vi "TEST_ProcessData.vi"() -> ()   [LabVIEW 2024]
doc: "This VI is used to test the Spec LUT (Look Up Table) Select ChA!ChB and Drain!Fill\nShould produce the spec index for the level entered.\nNote: Meausre shows the value whre Measure R is enabled."
uses:
  Control Definitions/Def FullCfg.ctl
  Control Definitions/Def BenchCfg.ctl
  Control Definitions/Def PumpCtlRefs.ctl
  Control Definitions/Def_PumpSpeed.ctl
  Control Definitions/Def Bench Status.ctl
  Control Definitions/Def_LevelSwitched.ctl
  Control Definitions/Def Spec RNG.ctl
  Control Definitions/Ded LUT_Status.ctl
  Control Definitions/Def Results2.ctl
  Control Definitions/Def_ATPStatus.ctl
panel:
  out "L Err Num":i32
  out "R Err Num":i32
  in  "ATP Check":bool
  out "Results out":T1 {"Resistor" format="%.1f"; "Drain" format="%.3f"; "Fill" format="%.3f"}
  out "element":T3={"Specs"=[8.5, 8.5, 0.0, 102.0, 98.0, 0.0, 0.0], "LUT Status"={"ChA/!ChB"=TRUE, "Drain/!Fill"=FALSE, "In Range?"=FALSE, "Switch Range?"=FALSE, "Measure R?"=FALSE, "Vaild R?"=FALSE, "Index(n)"=0, "Index(n)-1"=-1, "Index Max"=13, "Index(n-1)"=0}}
  out "Level Out":T5={"Switched"=FALSE, "Level OUt"=8.030499999999925, "Double Err"=FALSE}
  in  "Inputs":cluster{" Ohms":dbl, "Level OUt":dbl}={" Ohms"=101.0, "Level OUt"=8.030499999999925}
  in  "ChB!ChA":bool
  in  "Test Index":i32
  in  "Full Cfg 2":T6={"Bench Config"={"Name"="OLR001", {"Step Levels"=0.05, "Tolerance"=0.01, "Sample Rate"=0.05, "Resistor"=100.0, "M Level Cal"=1.0, "[B Level Cal"=0.0, "Max Fill Rate"=0.002, "Empty Inches"=8.0, "Full Inches"=2.6}}, "Test Value Table "=[[98.0, 102.0, 8.5, 8.5, 8.5, 8.5, 98.0, 102.0, 8.5, 8.5, 8.5, 8.5], [98.0, 102.0, 7.91, 8.01, 7.55, 7.65, 98.0, 102.0, 7.685, 7.785, 7.325, 7.425], [197.0, 203.0, 7.46, 7.56, 7.1, 7.2, 197.0, 203.0, 7.235, 7.335, 6.875, 6.975], [296.0, 304.0, 7.01, 7.11, 6.65, 6.75, 296.0, 304.0, 6.785, 6.885, 6.425, 6.525], [395.0, 405.0, 6.56, 6.66, 6.2, 6.3, 395.0, 405.0, 6.335, 6.435, 5.975, 6.075], [494.0, 506.0, 6.11, 6.21, 5.75, 5.85, 494.0, 506.0, 5.885, 5.985, 5.525, 5.625], [593.0, 607.0, 5.66, 5.76, 5.3, 5.4, 593.0, 607.0, 5.435, 5.535, 5.075, 5.175], [692.0, 708.0, 5.21, 5.31, 4.85, 4.95, 692.0, 708.0, 4.985, 5.085, 4.625, 4.725], [791.0, 809.0, 4.76, 4.86, 4.4, 4.5, 791.0, 809.0, 4.535, 4.635, 4.175, 4.275], [890.0, 910.0, 4.31, 4.41, 3.95, 4.05, 890.0, 910.0, 4.085, 4.185, 3.725, 3.825], [989.0, 1011.0, 3.86, 3.96, 3.5, 3.6, 989.0, 1011.0, 3.635, 3.735, 3.275, 3.375], [1088.0, 1112.0, 3.41, 3.51, 3.05, 3.15, 1088.0, 1112.0, 3.185, 3.285, 2.825, 2.925], [1088.0, 1112.0, 2.5, 2.5, 2.5, 2.5, 1088.0, 1112.0, 2.5, 2.5, 2.5, 2.5]], "Table Col Titles"=[["Aohm Lo", "Aohm Hi", "A Fill Lo", "A Fill Hi", "A Drain Lo", "A Drain Hi", "Bohm Lo", "Bohm Hi", "B Fill Lo", "B Fill Hi", "B Drain Lo", "B Drain Hi"]], "cluster"={"Fill "=refnum, "Drain"=refnum, "Level PV"=refnum, "Pump Speed"=refnum, "Run Test"=refnum, "Sim"=refnum, "Jog"=refnum, "Level SP"=refnum}, "Bench Status"={"Pump Status"=refnum, "Instrumnet\n Status"=refnum}}
  in  "stop":bool
  in  "Drain!Fill":bool
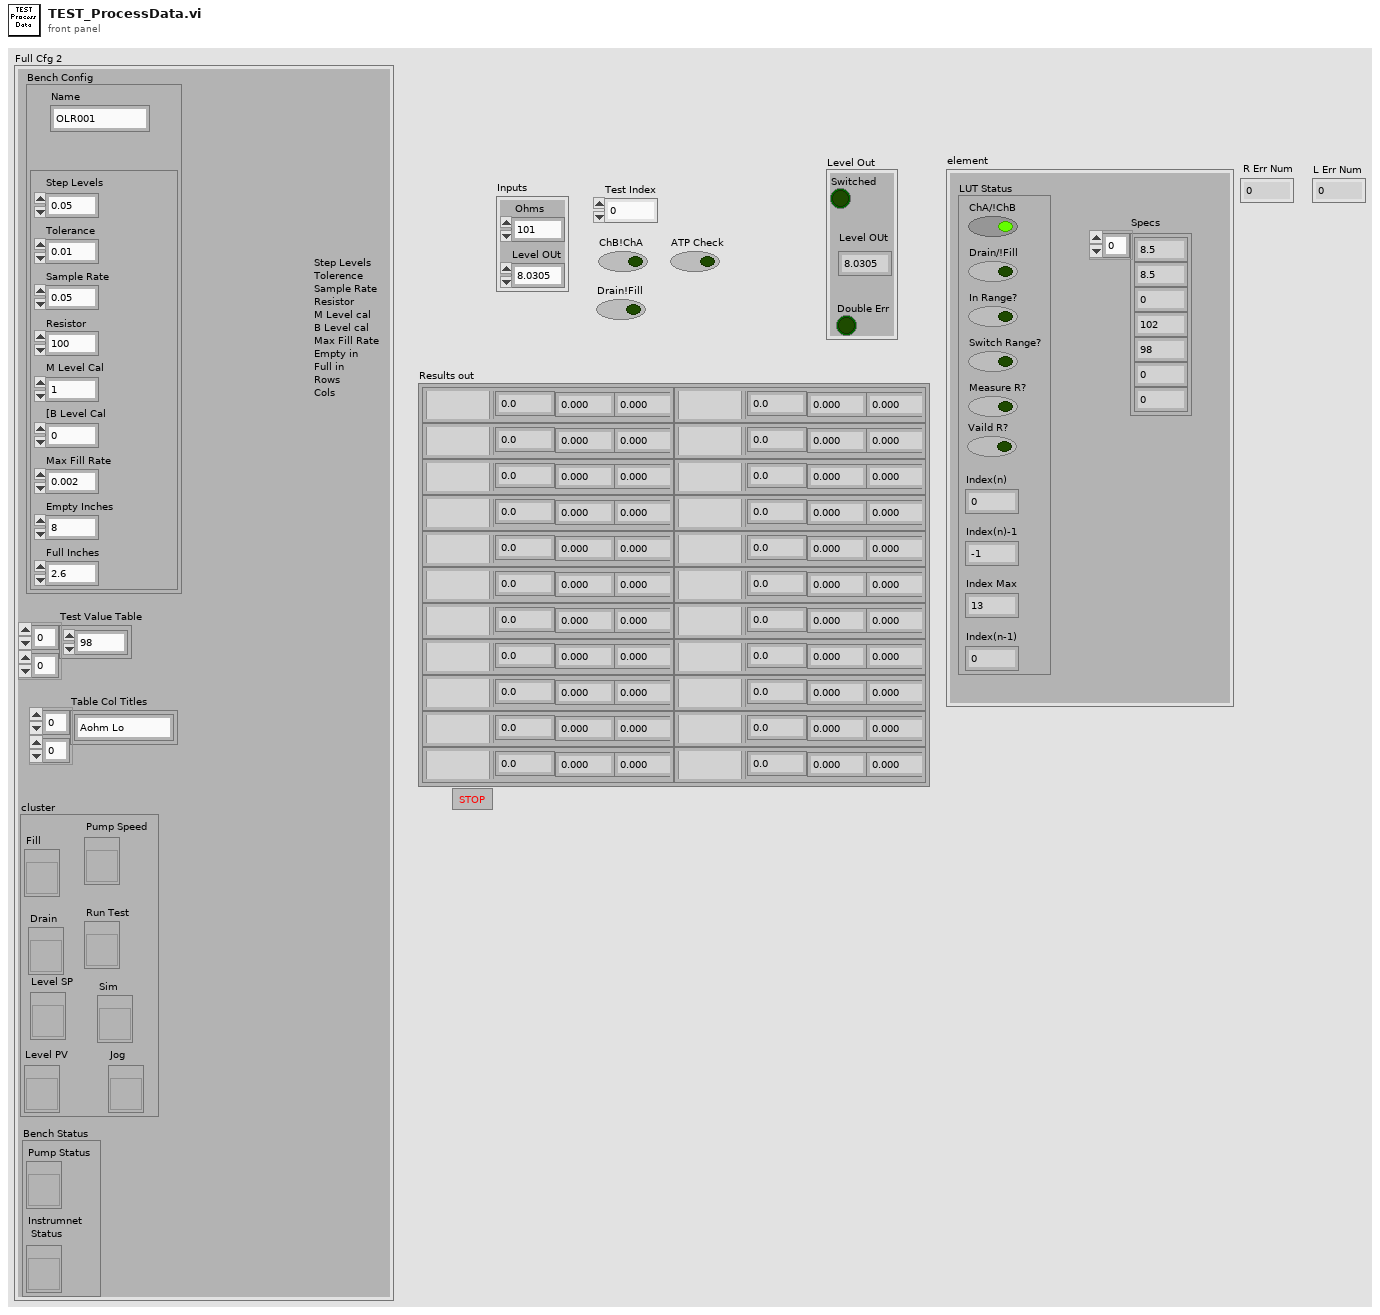
[diagram p1: front panel]
types:
  T1 = typedef "Def Results2.ctl" = cluster{"Fill":dbl, "Drain":dbl, "Status":T2, "Resistor":dbl}[][]
  T2 = typedef "Def_ATPStatus.ctl" = i16
  T3 = typedef "Def Spec RNG.ctl" = cluster{"Specs":dbl[], "LUT Status":T4}
  T4 = typedef "Ded LUT_Status.ctl" = cluster{"ChA/!ChB":bool, "Drain/!Fill":bool, "In Range?":bool, "Switch Range?":bool, "Measure R?":bool, "Vaild R?":bool, "Index(n)":i32, "Index(n)-1":i32, "Index Max":i32, "Index(n-1)":i32}
  T5 = typedef "Def_LevelSwitched.ctl" = cluster{"Switched":bool, "Level OUt":dbl, "Double Err":bool}
  T6 = typedef "Def FullCfg.ctl" = cluster{"Bench Config":T7, "Test Value Table ":dbl[][], "Table Col Titles":string[][], "cluster":T8, "Bench Status":T9}
  T7 = typedef "Def BenchCfg.ctl" = cluster{"Name":string, cluster{"Step Levels":dbl, "Tolerance":dbl, "Sample Rate":dbl, "Resistor":dbl, "M Level Cal":dbl, "[B Level Cal":dbl, "Max Fill Rate":dbl, "Empty Inches":dbl, "Full Inches":dbl}}
  T8 = typedef "Def PumpCtlRefs.ctl" = cluster{"Fill ":refnum<vi>, "Drain":refnum<vi>, "Level PV":refnum<vi>, "Pump Speed":refnum<vi>, "Run Test":refnum<vi>, "Sim":refnum<vi>, "Jog":refnum<vi>, "Level SP":refnum<vi>}
  T9 = typedef "Def Bench Status.ctl" = cluster{"Pump Status":refnum<vi>, "Instrumnet\n Status":refnum<vi>}
  T10 = cluster{"Fill":dbl, "Drain":dbl, "Status":T2, "Resistor":dbl}[]
  T11 = cluster{"Fill":dbl, "Drain":dbl, "Status":i16, "Resistor":dbl}[]
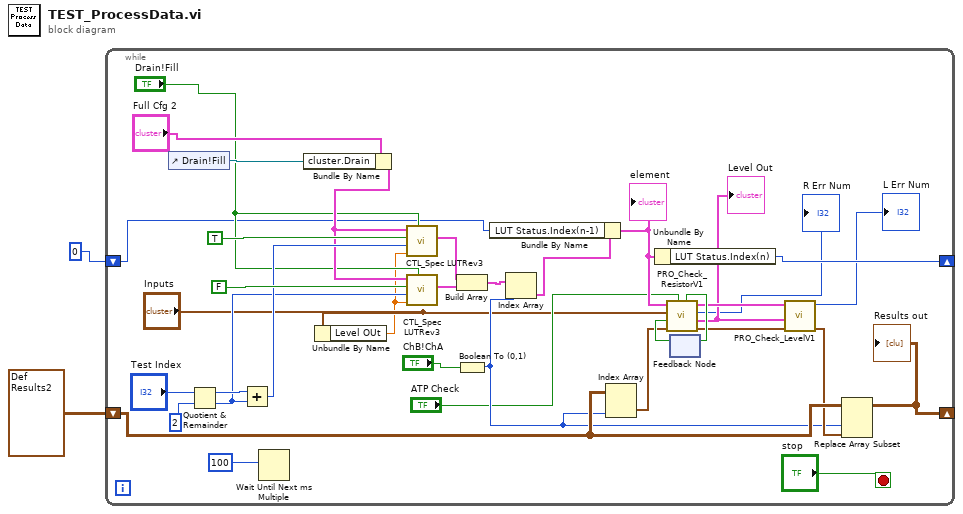
[diagram p0: block diagram]
diagram:
  n1 = while {
    shift-right: [w20] -> _
    shift-left: 0 ("Index(n)") -> [w17]
    shift-right: [w13] -> _
    shift-left: T1 [[{"Fill"=0.0, "Drain"=0.0, "Status"=0, "Resistor"=0.0}, {"Fill"=0.0, "Drain"=0.0, "Status"=0, "Resistor"=0.0}], [{"Fill"=0.0, "Drain"=0.0, "Status"=0, "Resistor"=0.0}, {"Fill"=0.0, "Drain"=0.0, "Status"=0, "Resistor"=0.0}], [{"Fill"=0.0, "Drain"=0.0, "Status"=0, "Resistor"=0.0}, {"Fill"=0.0, "Drain"=0.0, "Status"=0, "Resistor"=0.0}], [{"Fill"=0.0, "Drain"=0.0, "Status"=0, "Resistor"=0.0}, {"Fill"=0.0, "Drain"=0.0, "Status"=0, "Resistor"=0.0}], [{"Fill"=0.0, "Drain"=0.0, "Status"=0, "Resistor"=0.0}, {"Fill"=0.0, "Drain"=0.0, "Status"=0, "Resistor"=0.0}], [{"Fill"=0.0, "Drain"=0.0, "Status"=0, "Resistor"=0.0}, {"Fill"=0.0, "Drain"=0.0, "Status"=0, "Resistor"=0.0}], [{"Fill"=0.0, "Drain"=0.0, "Status"=0, "Resistor"=0.0}, {"Fill"=0.0, "Drain"=0.0, "Status"=0, "Resistor"=0.0}], [{"Fill"=0.0, "Drain"=0.0, "Status"=0, "Resistor"=0.0}, {"Fill"=0.0, "Drain"=0.0, "Status"=0, "Resistor"=0.0}], [{"Fill"=0.0, "Drain"=0.0, "Status"=0, "Resistor"=0.0}, {"Fill"=0.0, "Drain"=0.0, "Status"=0, "Resistor"=0.0}], [{"Fill"=0.0, "Drain"=0.0, "Status"=0, "Resistor"=0.0}, {"Fill"=0.0, "Drain"=0.0, "Status"=0, "Resistor"=0.0}], [{"Fill"=0.0, "Drain"=0.0, "Status"=0, "Resistor"=0.0}, {"Fill"=0.0, "Drain"=0.0, "Status"=0, "Resistor"=0.0}]] ("Results out") -> [w15]
    stop <- "stop" stop-if-true
    n2 = control-ref of="Drain!Fill"() -> (w38:refnum<vi>)
    n3 = Quotient & Remainder(x="Test Index", y=2) -> (x-y*floor(x/y)=w33:i32, floor(x/y)=w27:i32)
    n4 = Add(x=w33, y=w27) -> (x+y=w30:i32)
    n5 = Wait Until Next ms Multiple(millisecond multiple=u32 100) -> ()  [unwired: 1 out]
    n6 = Bundle By Name(cluster="Full Cfg 2", "cluster.Drain"=w38) -> (w26:T6)
    n7 = Unbundle By Name("Inputs") -> ("Level OUt"=w7:dbl)
    n8 = call "CTL_Spec LUTRev3.vi"("Drain!Fill"="Drain!Fill", "Level IN inches"=w7, "Index"=w30, "ChA/!ChB"=TRUE, "Full Cfg"=w26) -> ("Spec Range Out"=w29:T3)  [unwired: 3 in, 3 out]
    n9 = call "CTL_Spec LUTRev3.vi"("Drain!Fill"="Drain!Fill", "Level IN inches"=w7, "Index"=w27, "ChA/!ChB"=FALSE, "Full Cfg"=w26) -> ("Spec Range Out"=w28:T3)  [unwired: 3 in, 3 out]
    n10 = Build Array(w29, w28) -> (w10:T3[])
    n11 = Boolean To (0,1)(Boolean="ChB!ChA") -> (0, 1=w11:i16)
    n12 = Index Array(array=w10, index=w11) -> (element=w19:T3)
    n13 = Bundle By Name(cluster=w19, "LUT Status.Index(n-1)"=w17) -> (w18:T3)
    "element" <- w18
    n14 = Index Array(array=w15, index (col)=w11) -> (element=w6:T10)  [unwired: 1 in]
    n15 = Unbundle By Name(w18) -> ("LUT Status.Index(n)"=w20:i32)
    n16 = feedback #1() -> (w21:bool)  [unwired: 1 in]
    n17 = call "PRO_Check_ResistorV1.vi"("ATP Check"="ATP Check", "Results IN"=w6, "Switched In"=w21, "Inputs"="Inputs", "ChA Spec RNG In"=w18) -> ("results out"=w5:T11, "Level Out"=w12:T5, "Err Num"=→"R Err Num":i32, "ChA Spec RNG Out"=w16:T3, "Switched Out"=w22:bool)  [unwired: 2 in]
    "Level Out" <- w12
    n18 = feedback-in #1(w22) -> ()
    n19 = call "PRO_Check_LevelV1.vi"("Results In"=w5, "Level In"=w12, "ChA Spec RNG In"=w16) -> ("Results Out"=w14:T11, "Err Num"=→"L Err Num":i32)  [unwired: 5 in, 2 out]
    n20 = Replace Array Subset(array=w15, new element=w14, index (col)=w11) -> (w13:T1)  [unwired: 1 in]
    "Results out" <- w13
  }
